vi "Teleop.vi"(10 "Match Info":T1={"Autonomous Elapsed Seconds"=0.0, "TeleOp Elapsed Seconds"=0.0, "Disabled Elapsed Seconds"=0.0, "Visited Autonomous"=FALSE, "Visited TeleOp"=FALSE, "Visited Disabled"=FALSE, "Autonomous Settings"={"Autonomous Style"=enum."Independent", "VI Refnum"=refnum}}, 11 "Call Context":T2) -> ()   [LabVIEW 2015]
doc: "This VI is called for each TeleOp packet received from the DS where the robot is not disabled. It is often used to read from the joysticks and update I/O or to update setpoints for timed control loops. It should complete and return within 20 milliseconds or it may miss DS packets."
uses:
  <vilib>/Rock Robotics/WPI/DriverStation/WPI_DriverStationDerivedRobotMode.ctl
  <vilib>/Rock Robotics/WPI/DriverStation/WPI_DriverStationMatch Info.ctl
  Robot Global Data.vi
  900/Team900-VIs/Logitech/F510/F510-X.vi
  <vilib>/Rock Robotics/Network Tables/SD Write Numeric Array.vi
  900/Team900-VIs/Team900SwerveDrive/SwerveDriveFuse.vi
  900/TeleArm/ArmControlManual.vi
  900/Team900-VIs/Team900SwerveDrive/Team900SwerveDrive.lvlib
  900/TeleArm/ArcadeArmControl.vi
panel:
  in  "Fast Pivot":dbl=0.75 format="%#_13g"
  in  "Slow Pivot":dbl=0.5 format="%#_13g"
  in  "Max Wheel Speed":dbl=20000.0
  out "error out":errorcluster
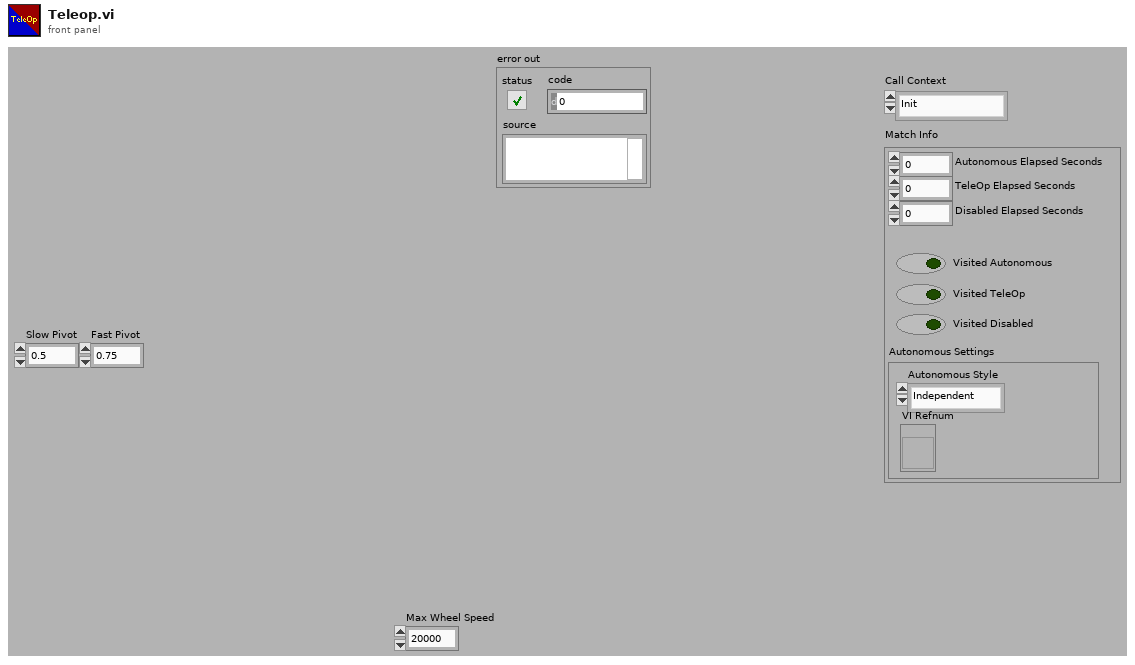
[diagram p1: front panel]
types:
  T1 = typedef "WPI_DriverStationMatch Info.ctl" = cluster{"Autonomous Elapsed Seconds":dbl, "TeleOp Elapsed Seconds":dbl, "Disabled Elapsed Seconds":dbl, "Visited Autonomous":bool, "Visited TeleOp":bool, "Visited Disabled":bool, "Autonomous Settings":cluster{"Autonomous Style":enum16{"Iterative", "Independent"}, "VI Refnum":refnum<vi>}}
  T2 = typedef "WPI_DriverStationDerivedRobotMode.ctl" = enum16{"Init", "Execute", "Stop"}
  T3 = cluster{"proportional gain (Kc)":dbl, "integral time (Ti, min)":dbl, "derivative time (Td, min)":dbl}
  T4 = cluster{"A":bool, "B":bool, "X":bool, "Y":bool, "LB":bool, "RB":bool, "Back":bool, "Start":bool, "LC":bool, "RC":bool, "LT":bool, "RT":bool}
  T5 = enum16{"Open", "Close", "Continue", "Stop", "Toggle"}
  T6 = typedef "WPI_MotorControlDeviceRef.ctl" = cluster{"DeviceStatus":errorcluster, "Type":T7, "PWM":cluster{"PWM Channel":T8, "DeadBand":T9}, "CAN":cluster{"Device Number":u8, "Control Mode":T10, "Semaphore":T11, "Max Vout":dbl, "TalonSRX Control Mode":T12}, "Invert":bool, "TransformRef":T13, "InvTransformRef":T13}
  T7 = typedef "WPI_MotorControlType.ctl" = enum16{"PWM", "CAN", "CANTalonSRX"}
  T8 = typedef "FPGA_DIOPWMChannel.ctl" = enum8{"PWM 0", "PWM 1", "PWM 2", "PWM 3", "PWM 4", "PWM 5", "PWM 6", "PWM 7", "PWM 8", "PWM 9", "PWM MXP 0", "PWM MXP 1", "PWM MXP 2", "PWM MXP 3", "PWM MXP 4", "PWM MXP 5", "PWM MXP 6", "PWM MXP 7", "PWM MXP 8", "PWM MXP 9", "Invalid"}
  T9 = typedef "WPI_PWMDeadband.ctl" = cluster{"Name":string, "maxPositivePwm":i32, "minPositivePwm":i32, "centerPwm":i32, "maxNegativePwm":i32, "minNegativePwm":i32, "angularRange":u16}
  T10 = typedef "WPI_CANJaguar_ControlMode.ctl" = enum8{"Percent VBus", "Current", "Speed", "Position", "Voltage"}
  T11 = typedef "Semaphore RefNum" = refnum<k1>
  T12 = typedef "WPI_CANTalonSRX_APIControlMode.ctl" = enum8{"Percent VBus", "Speed", "Position", "Slave", "Unchanged / Invalid"}
  T13 = typedef "WPI_PWMTransform_ConPane.ctl" = refnum<vi>
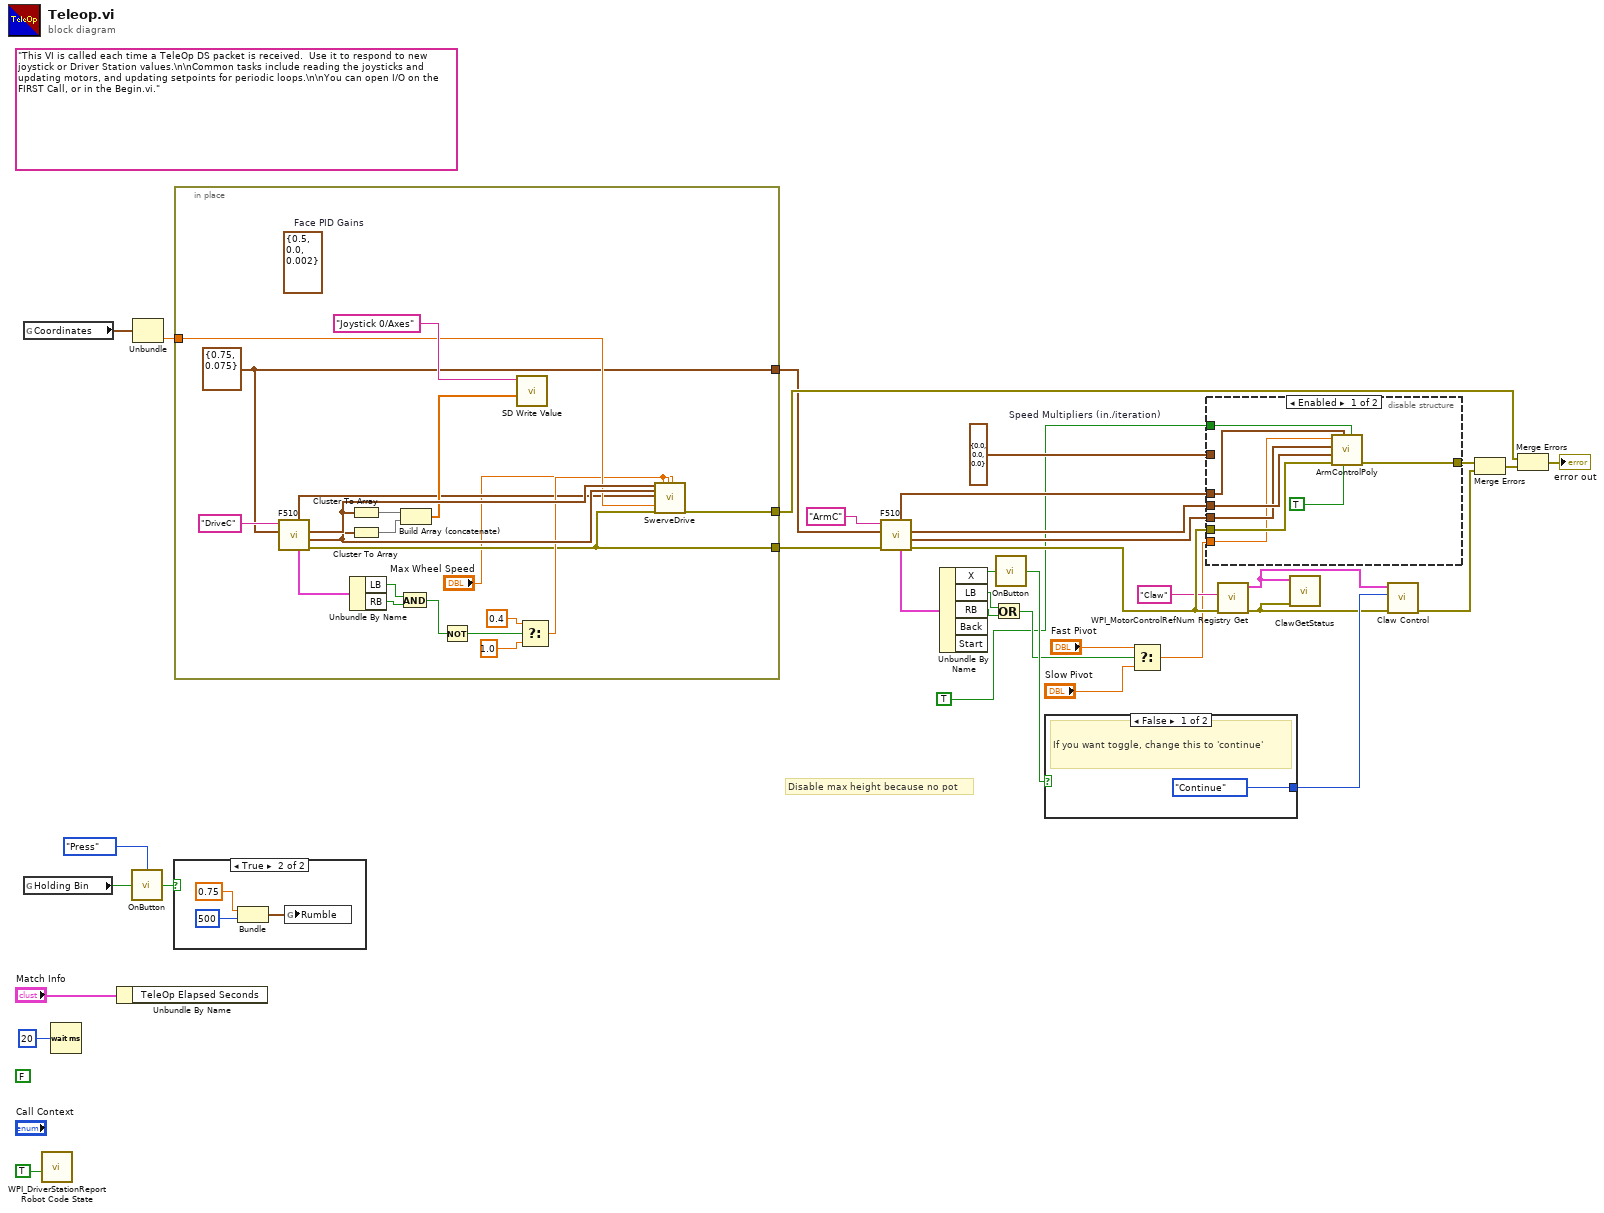
[diagram p0: block diagram]
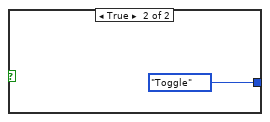
[diagram p3: hidden frame]
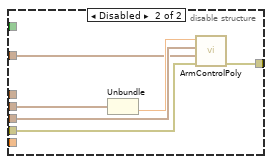
[diagram p4: hidden frame]
diagram:
  w21 = cluster{"X":dbl, "Y":dbl, "Wrist":dbl} {"X"=0.0, "Y"=0.0, "Wrist"=0.0}  # Speed Multipliers (in./iteration)
  (unwired) FALSE
  (unwired) "This VI is called each time a TeleOp DS packet is received.  Use it to respond to new joystick or Driver Station values.\n\nCommon tasks include reading the joysticks and updating motors, and updating setpoints for periodic loops.\n\nYou can open I/O on the FIRST Call, or in the Begin.vi."
  # "Disable max height because no pot"
  n1 = global read "Robot Global Data.vi" "Coordinates"() -> (w29:cluster{"X":dbl, "Y":dbl, "Heading":dbl})
  n2 = global read "Robot Global Data.vi" "Holding Bin"() -> (w12:bool)
  n3 = call <vilib>:"WPI_DriverStationReport Robot Code State.vi"("TeleOp"=TRUE ("Autonomous")) -> ()  [unwired: 10 in, 1 out]
  n4 = Wait (ms)(milliseconds to wait=u32 20) -> ()  [unwired: 1 out]
  n5 = Unbundle By Name("Match Info") -> ()  [unwired: 1 out]
  n6 = call "OnButton.vi"("Button"=w12, "Mode"=enum16{"Press", "Release", "Both"}."Press") -> ("Value"=w13:bool)
  n7 = Unbundle(w29) -> ("Heading"=w30:dbl)  [unwired: 2 out]
  n8 = case shown="True" w13 {
    frame False {
    }
    frame True {
      n9 = Bundle("t"=0.75, "f"=i16 500) -> (w36:cluster{"t":dbl, "f":i16})  [unwired: 1 in]
      n10 = global write "Robot Global Data.vi" "Rumble"(w36) -> ()
    }
  }
  n11 = in-place {
    in-place-border: w30 -> [w48]
    in-place-border: [w43] -> w33
    in-place-border: [w42] -> w31
    in-place-border: [w39] -> w28
    (unwired) T3 {"proportional gain (Kc)"=0.5, "integral time (Ti, min)"=0.0, "derivative time (Td, min)"=0.002}  # Face PID Gains
    w39 = cluster{"Scale":dbl, "Deadzone":dbl} {"Scale"=0.75, "Deadzone"=0.075} ("Deadzone Scale Cluster")
    n12 = call-poly "F510.vi"("Deadzone Scale Cluster"=w39, "refnum name"="DriveC") -> ("error out"=w43:errorcluster, "Right Stick"=w57:cluster{"X":dbl, "Y":dbl}, "Left Stick"=w58:cluster{"X":dbl, "Y":dbl}, "Buttons"=w50:T4, "Triggers"=w41:cluster{"Left":dbl, "Right":dbl})  [unwired: 3 in, 2 out]
    n13 = Unbundle By Name(w50) -> ("LB"=w52:bool, "RB"=w51:bool)
    n14 = Cluster To Array(cluster=w58) -> (array=w56:dbl[])
    n15 = Cluster To Array(cluster=w57) -> (array=w55:dbl[])
    n16 = And(x=w52, y=w51) -> (x .and. y?=w53:bool)
    n17 = Build Array (concatenate)(w56, w55) -> (w54:dbl[])
    n18 = Not(x=w53) -> (.not. x?=w45:bool)
    n19 = call-poly <vilib>:"SD Write Value.vi"("Numeric Array"=w54, "Name"="Joystick 0/Axes") -> ()  [unwired: 8 in, 2 out]
    n20 = Select(t=0.4 ("Slow Speed Multiplier"), s=w45, f=1.0 ("Default Speed Multiplier")) -> (s? t:f=w44:dbl)
    n21 = call-poly "SwerveDrive.vi"("Strafe Joystick Axes"=w58, "Face Joystick Axes"=w57, "Trigger Axes/Turn Speed"=w41, "Angle (degrees; 0 = right)"=w48, "error in (no error)"=w43, "Strafe Multiplier"=w44, "Rotation Multiplier"=w44, "Max Wheel Speed"="Max Wheel Speed") -> ("error out"=w42:errorcluster)  [unwired: 10 in, 1 out]
  }
  n22 = call-poly "F510.vi"("error in (no error)"=w33, "Deadzone Scale Cluster"=w28, "refnum name"="ArmC") -> ("error out"=w18:errorcluster, "Right Stick"=w22:cluster{"X":dbl, "Y":dbl}, "Left Stick"=w23:cluster{"X":dbl, "Y":dbl}, "Buttons"=w6:T4, "Triggers"=w24:cluster{"Left":dbl, "Right":dbl})  [unwired: 2 in, 2 out]
  n23 = Unbundle By Name(w6) -> ("X"=w9:bool, "LB"=w8:bool, "RB"=w7:bool)  [unwired: 2 out]
  n24 = Or(x=w8, y=w7) -> (x .or. y?=w10:bool)
  n25 = call "OnButton.vi"("Button"=w9) -> ("Value"=w16:bool)  [unwired: 1 in]
  n26 = case shown="False" w16 {
    tunnel: [T5."Continue" ("Operation") T5."Toggle" ("Operation")] -> w15
    frame False {
      # "If you want toggle, change this to 'continue'"
    }
    frame True {
    }
  }
  n27 = Select(t="Fast Pivot", s=w10, f="Slow Pivot") -> (s? t:f=w11:dbl)
  n28 = disable-structure shown="Enabled" {
    disable-tunnel: [w69 w74] -> w20
    disable-tunnel: w24 -> [w68 _]
    disable-tunnel: w23 -> [w66 w72]
    disable-tunnel: w22 -> [w65 w73]
    disable-tunnel: w18 -> [w67 w75]
    disable-tunnel: w21 -> [_ w70]
    disable-tunnel: w11 -> [w63 _]
    disable-tunnel: TRUE -> [w62 _]
    frame Enabled {
      n29 = call-poly "ArmControlPoly.vi"("Override Height Limit"=w62, "Wrist PID?"=TRUE, "Extension Triggers"=w68, "error in (no error)"=w67, "Pivot Stick"=w66, "Wrist Stick"=w65, "Pivot Multiplier"=w63) -> ("error out"=w69:errorcluster)  [unwired: 4 in]
    }
    frame Disabled {
      n30 = Unbundle(w72) -> ("Y"=w71:dbl)  [unwired: 1 out]
      n31 = call-poly "ArmControlPoly.vi"("error in (no error)"=w75, "Speed Multipliers"=w70, "X/Y Stick"=w73, "Wrist Stick"=w71) -> ("error out"=w74:errorcluster)  [unwired: 7 in]
    }
  }
  n32 = call <vilib>:"WPI_MotorControlRefNum Registry Get.vi"("error in (no error)"=w18, "refnum name"="Claw") -> ("error out"=w3:errorcluster, "MotorControlDevRef"=w2:T6)  [unwired: 8 in]
  n33 = call "ClawGetStatus.vi"("error in (no error)"=w3, "MotorControlDevRef"=w2) -> ()  [unwired: 5 in, 5 out]
  n34 = call "Claw Control.vi"("error in (no error)"=w3, "Operation"=w15, "MotorControlDevRef"=w2) -> ("error out"=w19:errorcluster)  [unwired: 3 in, 3 out]
  n35 = Merge Errors(w20, w19) -> (w27:errorcluster)
  n36 = Merge Errors(w31, w27) -> (→"error out":errorcluster)
